vi "Day 5 solution.vi"() -> ()   [LabVIEW 2020]
uses:
  day 5 - stack--cluster.ctl
  <vilib>/regexp/Match Regular Expression.xnode
panel:
  in  "Mover type":enum16{"1 crate mover", "Multicrate mover"}(ring)
  out "Top crates":string
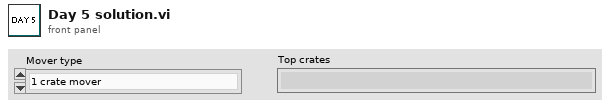
[diagram p1: front panel]
types:
  T1 = typedef "day 5 - stack--cluster.ctl" = cluster{"Crates":string[]}
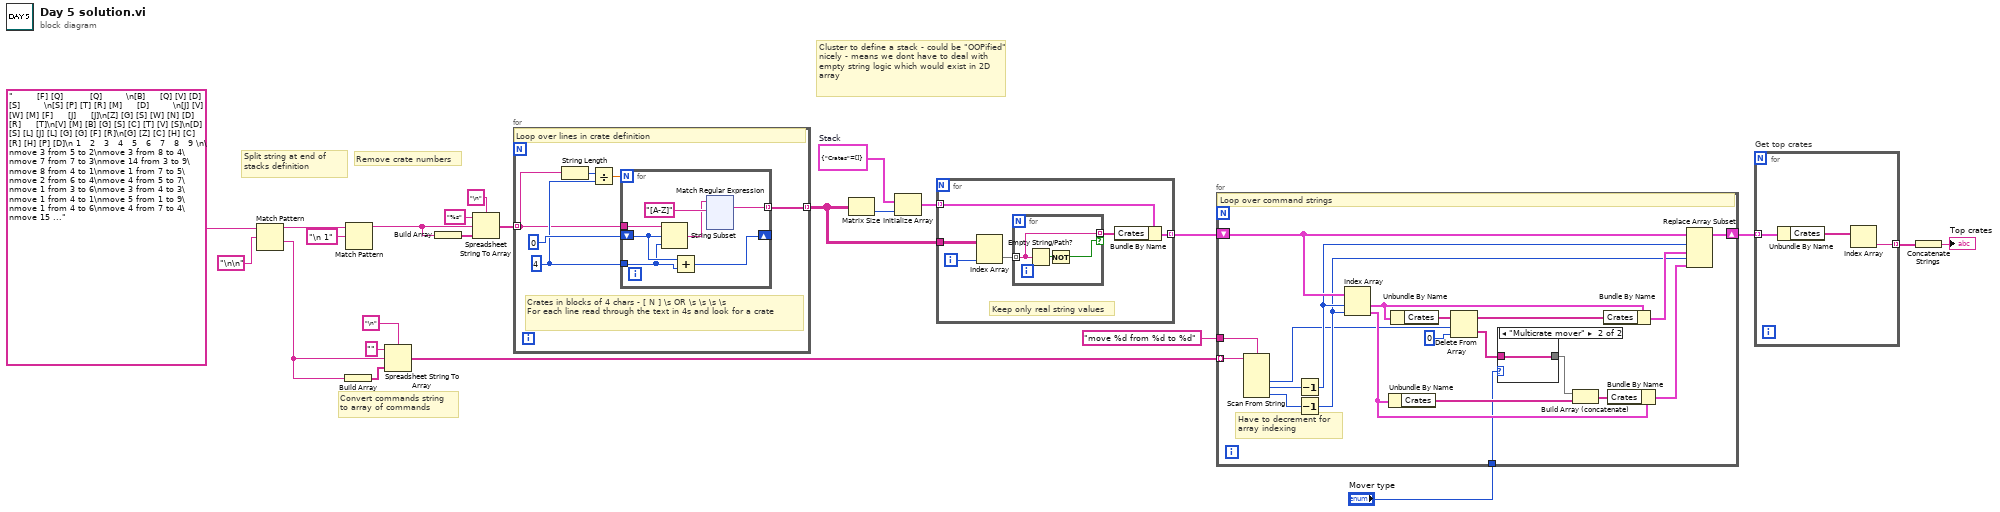
[diagram p0: block diagram]
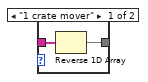
[diagram p2: hidden frame]
diagram:
  w22 = T1 {"Crates"=[]}  # Stack
  # "Convert commands string\nto array of commands"
  # "Cluster to define a stack - could be \"OOPified\" nicely - means we dont have to deal with empty string logic which would exist in 2D array"
  # "Remove crate numbers"
  # "Split string at end of stacks definition"
  n1 = Match Pattern(string="        [F] [Q]         [Q]        \n[B]     [Q] [V] [D]     [S]        \n[S] [P] [T] [R] [M]     [D]        \n[J] [V] [W] [M] [F]     [J]     [J]\n[Z] [G] [S] [W] [N] [D] [R]     [T]\n[V] [M] [B] [G] [S] [C] [T] [V] [S]\n[D] [S] [L] [J] [L] [G] [G] [F] [R]\n[G] [Z] [C] [H] [C] [R] [H] [P] [D]\n 1   2   3   4   5   6   7   8   9 \n\nmove 3 from 5 to 2\nmove 3 from 8 to 4\nmove 7 from 7 to 3\nmove 14 from 3 to 9\nmove 8 from 4 to 1\nmove 1 from 7 to 5\nmove 2 from 6 to 4\nmove 4 from 5 to 7\nmove 1 from 3 to 6\nmove 3 from 4 to 3\nmove 1 from 4 to 1\nmove 5 from 1 to 9\nmove 1 from 4 to 6\nmove 4 from 7 to 4\nmove 15 from 9 to 2\nmove 7 from 1 to 6\nmove 3 from 3 to 5\nmove 1 from 4 to 9\nmove 2 from 5 to 3\nmove 2 from 4 to 9\nmove 4 from 1 to 6\nmove 1 from 3 to 1\nmove 1 from 3 to 2\nmove 4 from 6 to 3\nmove 24 from 2 to 8\nmove 4 from 9 to 8\nmove 1 from 1 to 3\nmove 2 from 5 to 4\nmove 1 from 2 to 4\nmove 19 from 8 to 1\nmove 5 from 3 to 9\nmove 8 from 1 to 3\nmove 3 from 4 to 1\nmove 6 from 9 to 5\nmove 2 from 3 to 4\nmove 1 from 8 to 5\nmove 2 from 4 to 6\nmove 11 from 6 to 1\nmove 8 from 8 to 7\nmove 1 from 6 to 5\nmove 13 from 1 to 3\nmove 1 from 1 to 7\nmove 2 from 7 to 8\nmove 5 from 7 to 1\nmove 2 from 8 to 4\nmove 3 from 5 to 3\nmove 11 from 3 to 1\nmove 2 from 5 to 3\nmove 2 from 5 to 3\nmove 2 from 7 to 1\nmove 7 from 3 to 1\nmove 1 from 4 to 5\nmove 1 from 6 to 4\nmove 3 from 4 to 7\nmove 3 from 7 to 1\nmove 6 from 3 to 5\nmove 1 from 5 to 9\nmove 4 from 5 to 4\nmove 2 from 3 to 4\nmove 8 from 9 to 2\nmove 5 from 4 to 6\nmove 1 from 6 to 5\nmove 1 from 4 to 9\nmove 39 from 1 to 7\nmove 7 from 2 to 6\nmove 1 from 9 to 3\nmove 1 from 2 to 7\nmove 1 from 3 to 1\nmove 5 from 7 to 3\nmove 4 from 5 to 1\nmove 19 from 7 to 9\nmove 1 from 9 to 8\nmove 1 from 9 to 7\nmove 5 from 9 to 3\nmove 6 from 6 to 7\nmove 1 from 8 to 3\nmove 4 from 1 to 4\nmove 23 from 7 to 6\nmove 1 from 1 to 6\nmove 21 from 6 to 2\nmove 3 from 4 to 8\nmove 7 from 6 to 1\nmove 1 from 4 to 9\nmove 1 from 6 to 7\nmove 6 from 1 to 2\nmove 1 from 7 to 4\nmove 15 from 2 to 8\nmove 5 from 3 to 8\nmove 22 from 8 to 7\nmove 1 from 8 to 1\nmove 5 from 3 to 4\nmove 1 from 3 to 2\nmove 1 from 1 to 2\nmove 3 from 4 to 8\nmove 3 from 8 to 9\nmove 11 from 2 to 1\nmove 2 from 1 to 4\nmove 15 from 9 to 5\nmove 22 from 7 to 3\nmove 2 from 4 to 9\nmove 3 from 4 to 2\nmove 8 from 1 to 8\nmove 6 from 8 to 6\nmove 1 from 6 to 2\nmove 3 from 6 to 9\nmove 3 from 2 to 7\nmove 4 from 2 to 9\nmove 2 from 7 to 5\nmove 1 from 1 to 7\nmove 2 from 8 to 2\nmove 2 from 7 to 5\nmove 9 from 5 to 3\nmove 8 from 5 to 2\nmove 1 from 6 to 4\nmove 1 from 6 to 9\nmove 1 from 2 to 9\nmove 2 from 5 to 1\nmove 7 from 2 to 3\nmove 1 from 4 to 3\nmove 1 from 2 to 4\nmove 5 from 3 to 4\nmove 6 from 9 to 3\nmove 1 from 2 to 6\nmove 6 from 9 to 6\nmove 2 from 1 to 8\nmove 3 from 6 to 3\nmove 2 from 8 to 6\nmove 6 from 4 to 1\nmove 14 from 3 to 9\nmove 1 from 6 to 4\nmove 3 from 3 to 9\nmove 1 from 4 to 5\nmove 10 from 9 to 6\nmove 6 from 6 to 7\nmove 2 from 1 to 8\nmove 1 from 8 to 6\nmove 16 from 3 to 2\nmove 1 from 8 to 1\nmove 1 from 7 to 1\nmove 7 from 3 to 4\nmove 1 from 6 to 5\nmove 4 from 2 to 3\nmove 5 from 4 to 9\nmove 2 from 4 to 5\nmove 4 from 7 to 4\nmove 5 from 9 to 6\nmove 2 from 5 to 4\nmove 11 from 6 to 7\nmove 1 from 6 to 8\nmove 5 from 1 to 5\nmove 2 from 6 to 4\nmove 7 from 7 to 3\nmove 1 from 8 to 6\nmove 2 from 7 to 3\nmove 1 from 1 to 3\nmove 3 from 2 to 8\nmove 9 from 2 to 5\nmove 1 from 6 to 1\nmove 1 from 4 to 8\nmove 7 from 4 to 7\nmove 8 from 5 to 6\nmove 1 from 7 to 2\nmove 1 from 7 to 4\nmove 3 from 7 to 8\nmove 1 from 2 to 3\nmove 1 from 1 to 2\nmove 1 from 1 to 7\nmove 3 from 7 to 6\nmove 11 from 6 to 2\nmove 4 from 8 to 7\nmove 2 from 8 to 7\nmove 15 from 3 to 2\nmove 7 from 9 to 4\nmove 3 from 3 to 2\nmove 4 from 4 to 7\nmove 5 from 7 to 3\nmove 3 from 4 to 6\nmove 3 from 6 to 9\nmove 1 from 4 to 2\nmove 1 from 8 to 1\nmove 2 from 3 to 7\nmove 2 from 3 to 7\nmove 23 from 2 to 5\nmove 1 from 9 to 1\nmove 1 from 7 to 9\nmove 1 from 1 to 8\nmove 8 from 7 to 1\nmove 1 from 8 to 4\nmove 1 from 4 to 2\nmove 3 from 9 to 8\nmove 1 from 7 to 9\nmove 22 from 5 to 9\nmove 1 from 8 to 5\nmove 1 from 7 to 4\nmove 1 from 4 to 5\nmove 1 from 8 to 3\nmove 2 from 9 to 3\nmove 5 from 5 to 2\nmove 5 from 5 to 4\nmove 3 from 2 to 7\nmove 1 from 7 to 3\nmove 6 from 1 to 7\nmove 4 from 3 to 1\nmove 6 from 2 to 8\nmove 1 from 5 to 6\nmove 2 from 8 to 1\nmove 12 from 9 to 4\nmove 8 from 9 to 4\nmove 1 from 2 to 9\nmove 2 from 9 to 8\nmove 3 from 2 to 8\nmove 5 from 8 to 6\nmove 7 from 7 to 1\nmove 4 from 8 to 9\nmove 1 from 6 to 1\nmove 17 from 4 to 7\nmove 1 from 2 to 4\nmove 2 from 4 to 1\nmove 6 from 4 to 6\nmove 1 from 1 to 4\nmove 7 from 1 to 5\nmove 9 from 7 to 9\nmove 8 from 9 to 8\nmove 5 from 8 to 3\nmove 1 from 5 to 6\nmove 2 from 3 to 6\nmove 1 from 9 to 1\nmove 1 from 6 to 1\nmove 10 from 6 to 1\nmove 1 from 5 to 1\nmove 2 from 9 to 1\nmove 1 from 9 to 7\nmove 2 from 6 to 8\nmove 2 from 8 to 2\nmove 1 from 6 to 8\nmove 22 from 1 to 9\nmove 9 from 7 to 5\nmove 1 from 8 to 1\nmove 2 from 8 to 3\nmove 4 from 5 to 9\nmove 1 from 8 to 3\nmove 5 from 1 to 9\nmove 2 from 7 to 3\nmove 2 from 4 to 7\nmove 1 from 8 to 5\nmove 2 from 2 to 4\nmove 1 from 5 to 8\nmove 9 from 5 to 8\nmove 2 from 7 to 5\nmove 2 from 4 to 5\nmove 3 from 8 to 4\nmove 3 from 4 to 3\nmove 2 from 8 to 6\nmove 1 from 6 to 4\nmove 3 from 5 to 9\nmove 1 from 6 to 3\nmove 12 from 3 to 5\nmove 1 from 3 to 1\nmove 7 from 5 to 4\nmove 1 from 1 to 3\nmove 1 from 8 to 1\nmove 7 from 5 to 1\nmove 6 from 9 to 6\nmove 29 from 9 to 5\nmove 2 from 4 to 6\nmove 26 from 5 to 2\nmove 24 from 2 to 7\nmove 1 from 3 to 2\nmove 8 from 1 to 7\nmove 7 from 6 to 9\nmove 2 from 5 to 3\nmove 1 from 6 to 4\nmove 3 from 8 to 5\nmove 2 from 3 to 8\nmove 2 from 2 to 8\nmove 5 from 9 to 2\nmove 27 from 7 to 2\nmove 2 from 8 to 3\nmove 2 from 9 to 5\nmove 3 from 8 to 5\nmove 2 from 7 to 4\nmove 3 from 4 to 7\nmove 2 from 3 to 2\nmove 4 from 5 to 1\nmove 5 from 7 to 2\nmove 29 from 2 to 8\nmove 9 from 8 to 3\nmove 2 from 4 to 8\nmove 7 from 3 to 2\nmove 3 from 5 to 4\nmove 1 from 7 to 5\nmove 3 from 5 to 6\nmove 2 from 1 to 8\nmove 2 from 6 to 8\nmove 3 from 4 to 2\nmove 4 from 4 to 2\nmove 1 from 6 to 8\nmove 8 from 2 to 4\nmove 2 from 3 to 5\nmove 1 from 4 to 1\nmove 3 from 1 to 2\nmove 4 from 8 to 2\nmove 3 from 4 to 9\nmove 3 from 4 to 1\nmove 2 from 9 to 5\nmove 1 from 4 to 6\nmove 4 from 5 to 1\nmove 1 from 6 to 8\nmove 1 from 9 to 3\nmove 4 from 2 to 3\nmove 15 from 8 to 2\nmove 9 from 8 to 1\nmove 1 from 3 to 9\nmove 5 from 1 to 9\nmove 3 from 9 to 7\nmove 2 from 7 to 6\nmove 3 from 3 to 2\nmove 1 from 7 to 8\nmove 1 from 9 to 6\nmove 1 from 9 to 8\nmove 2 from 8 to 2\nmove 1 from 1 to 2\nmove 1 from 3 to 7\nmove 4 from 1 to 7\nmove 19 from 2 to 5\nmove 1 from 1 to 4\nmove 1 from 7 to 4\nmove 1 from 1 to 5\nmove 3 from 1 to 4\nmove 1 from 1 to 8\nmove 6 from 2 to 4\nmove 7 from 2 to 1\nmove 2 from 7 to 9\nmove 8 from 2 to 8\nmove 2 from 7 to 3\nmove 1 from 6 to 4\nmove 10 from 4 to 6\nmove 5 from 6 to 7\nmove 2 from 9 to 8\nmove 6 from 8 to 9\nmove 1 from 2 to 3\nmove 2 from 8 to 3\nmove 5 from 1 to 8\nmove 8 from 5 to 2\nmove 8 from 8 to 7\nmove 7 from 2 to 8\nmove 1 from 1 to 2\nmove 1 from 9 to 7\nmove 1 from 4 to 2\nmove 2 from 2 to 6\nmove 5 from 9 to 3\nmove 2 from 8 to 6\nmove 2 from 3 to 9\nmove 4 from 8 to 6\nmove 7 from 6 to 1\nmove 8 from 1 to 5\nmove 1 from 8 to 7\nmove 1 from 9 to 6\nmove 12 from 5 to 3\nmove 1 from 4 to 8\nmove 2 from 9 to 5\nmove 1 from 2 to 3\nmove 3 from 5 to 1\nmove 1 from 1 to 5\nmove 21 from 3 to 8\nmove 2 from 1 to 5\nmove 6 from 5 to 7\nmove 2 from 5 to 6\nmove 10 from 6 to 9\nmove 1 from 6 to 8\nmove 13 from 8 to 2\nmove 2 from 5 to 4\nmove 2 from 4 to 3\nmove 4 from 9 to 1\nmove 5 from 7 to 8\nmove 12 from 8 to 1\nmove 5 from 9 to 6\nmove 1 from 3 to 7\nmove 2 from 6 to 5\nmove 11 from 2 to 1\nmove 1 from 8 to 4\nmove 16 from 1 to 9\nmove 1 from 2 to 6\nmove 1 from 8 to 5\nmove 12 from 9 to 3\nmove 14 from 7 to 2\nmove 1 from 7 to 9\nmove 1 from 4 to 2\nmove 1 from 7 to 5\nmove 3 from 9 to 5\nmove 4 from 6 to 9\nmove 3 from 9 to 4\nmove 1 from 8 to 4\nmove 2 from 4 to 5\nmove 1 from 7 to 1\nmove 5 from 3 to 5\nmove 2 from 4 to 2\nmove 8 from 2 to 7\nmove 7 from 2 to 4\nmove 1 from 3 to 7\nmove 3 from 9 to 7\nmove 2 from 2 to 9\nmove 3 from 4 to 5\nmove 6 from 1 to 8\nmove 6 from 1 to 5\nmove 3 from 9 to 2\nmove 22 from 5 to 9\nmove 1 from 5 to 6\nmove 2 from 2 to 3\nmove 5 from 7 to 6\nmove 5 from 8 to 9\nmove 2 from 7 to 2\nmove 20 from 9 to 4\nmove 1 from 8 to 3\nmove 2 from 2 to 5\nmove 1 from 2 to 5\nmove 15 from 4 to 8\nmove 1 from 5 to 7\nmove 6 from 9 to 1\nmove 5 from 4 to 8\nmove 2 from 4 to 8\nmove 1 from 2 to 1\nmove 5 from 6 to 5\nmove 5 from 5 to 7\nmove 1 from 9 to 8\nmove 5 from 7 to 2\nmove 2 from 5 to 1\nmove 4 from 7 to 5\nmove 1 from 5 to 9\nmove 1 from 6 to 8\nmove 1 from 7 to 2\nmove 6 from 3 to 4\nmove 3 from 5 to 7\nmove 1 from 9 to 2\nmove 6 from 2 to 3\nmove 1 from 3 to 4\nmove 13 from 8 to 9\nmove 7 from 1 to 5\nmove 6 from 9 to 2\nmove 1 from 1 to 4\nmove 6 from 2 to 3\nmove 1 from 1 to 4\nmove 5 from 9 to 7\nmove 11 from 8 to 4\nmove 7 from 7 to 3\nmove 2 from 7 to 8\nmove 1 from 8 to 2\nmove 8 from 4 to 1\nmove 2 from 1 to 6\nmove 2 from 5 to 8\nmove 3 from 1 to 9\nmove 1 from 8 to 2\nmove 11 from 3 to 2\nmove 2 from 8 to 9\nmove 9 from 4 to 7\nmove 11 from 3 to 8\nmove 7 from 9 to 6\nmove 5 from 4 to 6\nmove 3 from 7 to 3\nmove 1 from 7 to 1\nmove 5 from 7 to 6\nmove 2 from 3 to 5\nmove 1 from 3 to 4\nmove 5 from 2 to 5\nmove 1 from 1 to 7\nmove 1 from 4 to 8\nmove 1 from 7 to 6\nmove 7 from 5 to 7\nmove 2 from 5 to 7\nmove 3 from 1 to 7\nmove 1 from 2 to 3\nmove 1 from 6 to 4\nmove 1 from 3 to 4\nmove 1 from 5 to 3\nmove 18 from 6 to 4\nmove 9 from 7 to 1\nmove 14 from 4 to 6\nmove 3 from 6 to 4\nmove 12 from 6 to 7\nmove 2 from 5 to 3\nmove 3 from 7 to 4\nmove 6 from 4 to 7\nmove 5 from 1 to 7\nmove 5 from 4 to 5\nmove 5 from 2 to 1\nmove 9 from 8 to 4\nmove 9 from 1 to 3\nmove 2 from 8 to 2\nmove 4 from 2 to 4\nmove 1 from 7 to 6\nmove 1 from 2 to 3\nmove 1 from 8 to 9\nmove 1 from 6 to 9\nmove 2 from 9 to 3\nmove 3 from 4 to 1\nmove 13 from 3 to 5\nmove 12 from 5 to 1\nmove 7 from 1 to 8\nmove 1 from 3 to 6\nmove 4 from 5 to 4\nmove 1 from 5 to 2\nmove 8 from 4 to 9", regular expression="\n\n") -> (before substring=w10:string, after substring=w20:string)  [unwired: 1 in, 2 out]
  n2 = Build Array(w20) -> (w19:string[])
  n3 = Match Pattern(string=w10, regular expression="\n 1") -> (before substring=w6:string)  [unwired: 1 in, 3 out]
  n4 = Spreadsheet String To Array(delimiter (Tab)="\n", format string="", spreadsheet string=w20, array type (2D Dbl)=w19) -> (array=w16:string[])
  n5 = Build Array(w6) -> (w5:string[])
  n6 = Spreadsheet String To Array(delimiter (Tab)="\n", format string="%s", spreadsheet string=w6, array type (2D Dbl)=w5) -> (array=w4:string[])
  n7 = for {
    tunnel: w4 -> [w25] mode=indexing
    tunnel: [w29] -> w2 mode=indexing
    w28 = 4 ("length (rest)")
    # "Crates in blocks of 4 chars - [ N ] \\s OR \\s \\s \\s \\s\nFor each line read through the text in 4s and look for a crate"
    # "Loop over lines in crate definition"
    n8 = String Length(string=w25) -> (length=w27:i32)
    n9 = Divide(x=w27, y=w28) -> (x/y=w26:dbl)
    n10 = for {
      N: w26 -> [_]
      tunnel: w25 -> [w37]
      shift-right: [w34] -> _
      shift-left: 0 -> [w36]
      tunnel: w28 -> [w35]
      tunnel: [w32] -> w29 mode=indexing
      n11 = String Subset(string=w37, offset (0)=w36, length (rest)=w35) -> (substring=w31:string)
      n12 = Add(x=w36, y=w35) -> (x+y=w34:i32)
      n13 = xnode "Match Regular Expression"("input string"=w31, "regular expression"="[A-Z]") -> ("whole match"=w32:string)  [unwired: 4 in, 4 out]
    }
  }
  n14 = Matrix Size(0:w2) -> (2:w3:i32)  [unwired: 1 out]
  n15 = Initialize Array(w22, w3) -> (w21:T1[])
  n16 = for {
    tunnel: w2 -> [w157]
    tunnel: w21 -> [w154] mode=indexing
    tunnel: [w152] -> w15 mode=indexing
    i -> [w156]
    # "Keep only real string values"
    n17 = Index Array(array=w157, index (col)=w156) -> (element=w155:string[])  [unwired: 1 in]
    n18 = for {
      tunnel: w155 -> [w158] mode=indexing
      tunnel: [w158] -> w153 mode=indexing if=w159
      n19 = Empty String/Path?(string/path=w158) -> (empty?=w160:bool)
      n20 = Not(x=w160) -> (.not. x?=w159:bool)
    }
    n21 = Bundle By Name(cluster=w154, "Crates"=w153) -> (w152:T1)
  }
  n22 = for {
    tunnel: w16 -> [w181] mode=indexing
    shift-right: [w171] -> w13
    shift-left: w15 -> [w172]
    tunnel: "move %d from %d to %d" ("format string") -> [w180]
    tunnel: "Mover type" -> [w161]
    # "Have to decrement for \narray indexing"
    # "Loop over command strings"
    n23 = Scan From String(format string=w180, input string=w181) -> (output 1=w164:i32, output 2=w170:i32, output 3=w167:i32)  [unwired: 5 in, 3 out]
    n24 = Decrement(x=w170) -> (x-1=w166:i32)
    n25 = Decrement(x=w167) -> (x-1=w165:i32)
    n26 = Index Array(array=w172, index #1=w166, index #2=w165) -> (element #1=w177:T1, element #2=w175:T1)
    n27 = Unbundle By Name(w175) -> ("Crates"=w173:string[])
    n28 = Unbundle By Name(w177) -> ("Crates"=w179:string[])
    n29 = Delete From Array(array=w179, length=w164, index=0) -> (deleted portion=w163:string[], array with subset deleted=w176:string[])
    n30 = case shown="\"Multicrate mover\"" w161 {
      tunnel: w163 -> [w183 w184]
      tunnel: [w182 w184] -> w162
      frame "1 crate mover" {
        n31 = Reverse 1D Array(array=w183) -> (reversed array=w182:string[])
      }
      frame "Multicrate mover" {
      }
    }
    n32 = Build Array (concatenate)(w162, w173) -> (w174:string[])
    n33 = Bundle By Name(cluster=w177, "Crates"=w176) -> (w169:T1)
    n34 = Bundle By Name(cluster=w175, "Crates"=w174) -> (w168:T1)
    n35 = Replace Array Subset(array=w172, new element #1=w169, index #1=w166, new element #2=w168, index #2=w165) -> (w171:T1[])
  }
  n36 = for "Get top crates" {
    tunnel: w13 -> [w187] mode=indexing
    tunnel: [w185] -> w12 mode=indexing
    n37 = Unbundle By Name(w187) -> ("Crates"=w186:string[])
    n38 = Index Array(array=w186) -> (element=w185:string)  [unwired: 1 in]
  }
  n39 = Concatenate Strings(w12) -> (→"Top crates":string)
